vi "OKO PM100D-LV2017.vi"() -> ()   [LabVIEW 2017]
panel:
  out "Power":dbl format="%#_6e"
  out "Waveform Chart":dbl(graph)
  out "error out":errorcluster
  in  "stop":bool
  in  "Wavelength (0.0)":dbl=783.0
  in  "resource name":refnum<visa-resource-name>="USB0::0x1313::0x807B::400621::INSTR"
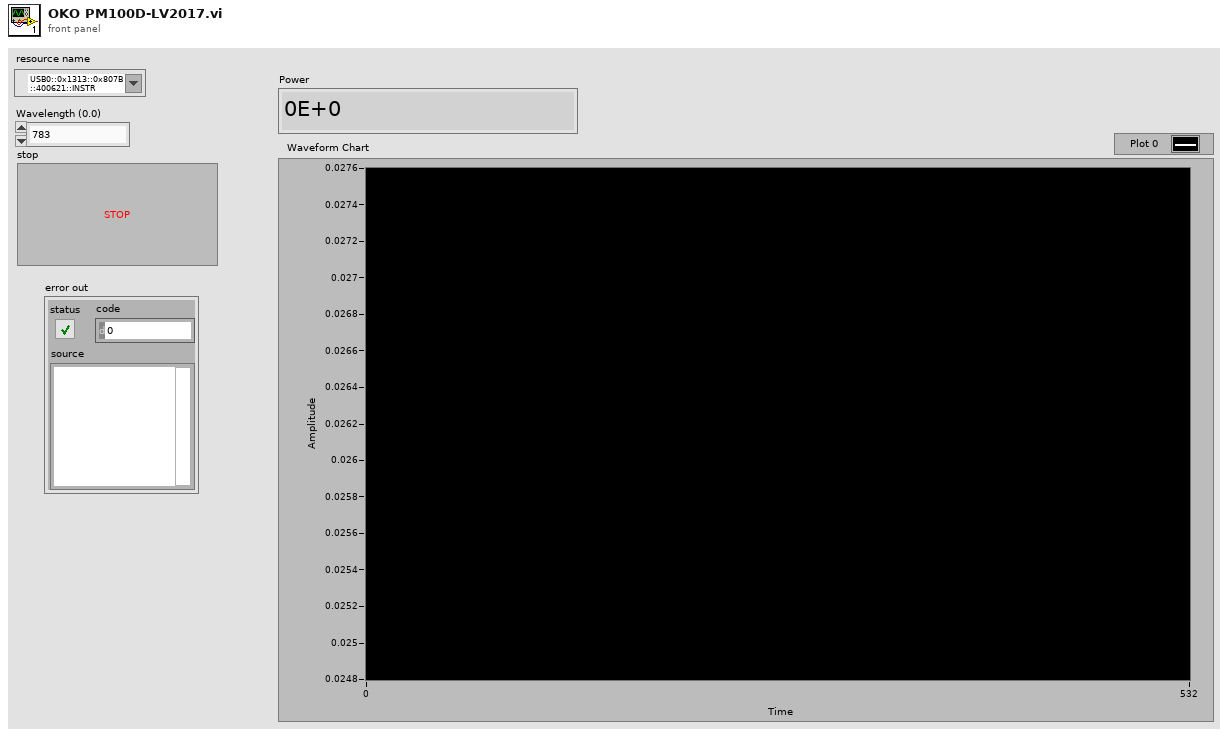
[diagram p1: front panel]
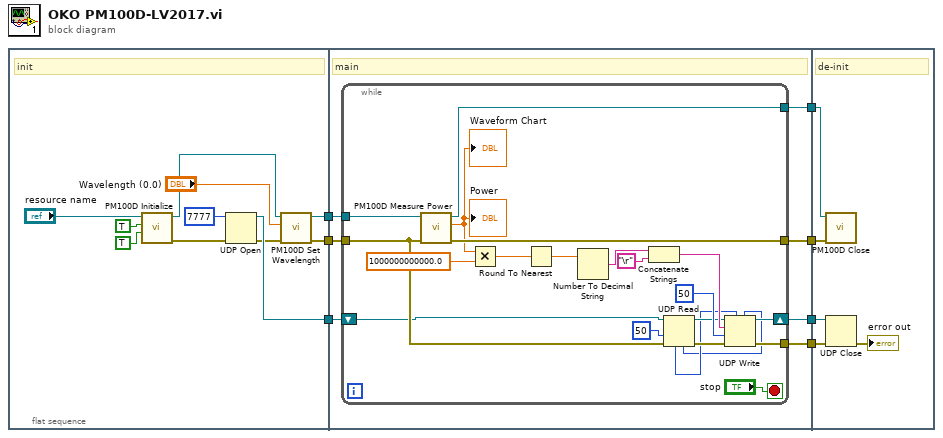
[diagram p0: block diagram]
diagram:
  n1 = flat-sequence {
    tunnel: [w14] -> w7
    tunnel: [w13] -> w6
    tunnel: [w10] -> w4
    tunnel: w7 -> [w23]
    tunnel: w6 -> [w22]
    tunnel: [w21] -> w5
    tunnel: w4 -> [w25]
    tunnel: [w24] -> w3
    tunnel: [w20] -> w2
    tunnel: [w19] -> w1
    tunnel: w5 -> [w51]
    tunnel: w3 -> [w50]
    tunnel: w2 -> [w48]
    tunnel: w1 -> [w47]
    frame #0 {
      # "init"
      n2 = call <instrlib>:"PM100D Initialize.vi"("Reset Device (Reset Device)"=TRUE, "ID Query (Do Query)"=TRUE, "resource name"="resource name") -> ("error out"=w9:errorcluster, "instrument handle out"=w15:refnum<visa-resource-name>)  [unwired: 7 in]
      n3 = UDP Open(8:w9, 11:u16 7777 ("port")) -> (port=w10:refnum<k16>, 0:w8:errorcluster)  [unwired: 3 in, 1 out]
      n4 = call <instrlib>:"PM100D Set Wavelength.vi"("error in (no error)"=w8, "Wavelength (0.0)"="Wavelength (0.0)", "instrument handle"=w15) -> ("error out"=w13:errorcluster, "instrument handle out"=w14:refnum<visa-resource-name>)  [unwired: 7 in]
    }
    frame #1 {
      # "main"
      n5 = while {
        shift-right: [w46] -> w24
        shift-left: w25 -> [w29]
        tunnel: w23 -> [w45]
        tunnel: w22 -> [w31]
        tunnel: [w44] -> w21
        tunnel: [w39] -> w20
        tunnel: [w38] -> w19
        stop <- "stop" stop-if-true
        n6 = call <instrlib>:"PM100D Measure Power.vi"("error in (no error)"=w31, "instrument handle"=w45) -> ("error out"=w39:errorcluster, "Power"=w34:dbl, "instrument handle out"=w44:refnum<visa-resource-name>)  [unwired: 7 in]
        "Waveform Chart" <- w34
        "Power" <- w34
        n7 = Multiply(x=w34, y=1000000000000.0) -> (x*y=w36:dbl)
        n8 = Round To Nearest(number=w36) -> (nearest integer value=w43:dbl)
        n9 = Number To Decimal String(number=w43) -> (decimal integer string=w35:string)  [unwired: 1 in]
        n10 = Concatenate Strings(w35, "\r") -> (w33:string)
        n11 = UDP Read(connection ID=w29, timeout ms (25000)=50, 8:w31) -> (error out=w30:errorcluster, 3:w28:refnum<k16>, 4:w26:u16, 6:w27:u32)  [unwired: 1 in, 1 out]
        n12 = UDP Write(address=w27, port or service name=w26, connection ID=w28, data in=w33, 8:w30, 9:50 ("timeout ms (25000)")) -> (error out=w38:errorcluster, 3:w46:refnum<k16>)
      }
    }
    frame #2 {
      # "de-init"
      n13 = call <instrlib>:"PM100D Close.vi"("error in (no error)"=w48, "instrument handle"=w51) -> ()  [unwired: 9 in, 1 out]
      n14 = UDP Close(connection ID=w50, 8:w47) -> (error out=→"error out":errorcluster)  [unwired: 1 out]
    }
  }
